vi "PI Measurement Type String Info.vi"(11 "Prompt Measurement Type String":string) -> (0 "Enumerations":string[](array[string]), 1 "Default Value":string, 2 "Is Enum?":bool, 3 "Is Scalar?":bool, 4 "comma list":string, 5 "Units (Scalar)":string)   [LabVIEW 2011]
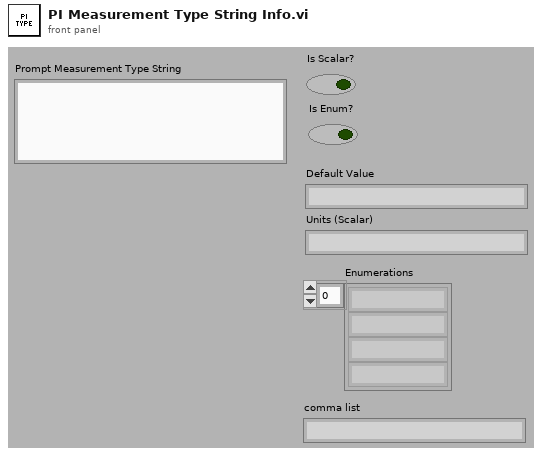
[diagram p1: front panel]
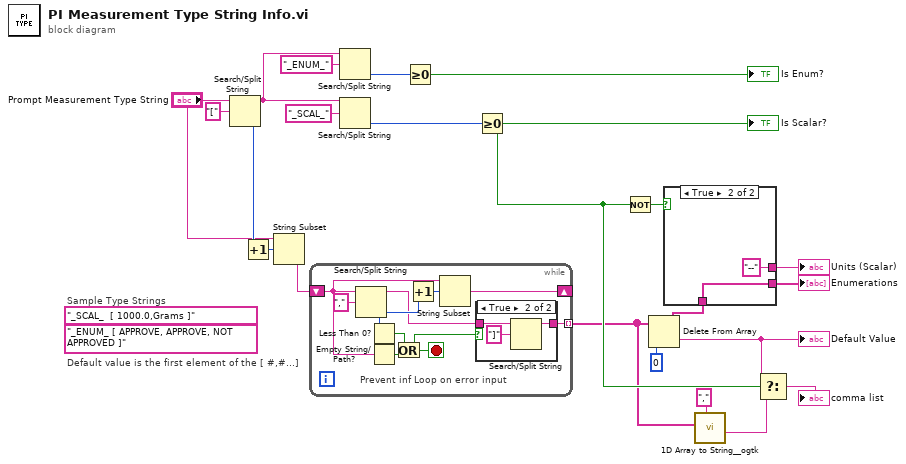
[diagram p0: block diagram]
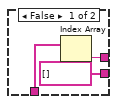
[diagram p2: hidden frame]
diagram:
  (unwired) "_ENUM_ [ APPROVE, APPROVE, NOT APPROVED ]" ("Name")
  (unwired) "_SCAL_  [ 1000.0,Grams ]" ("Name")
  # "Default value is the first element of the [ #,#...]"
  # "Sample Type Strings"
  n1 = Search/Split String(string="Prompt Measurement Type String", search string/char (-)="[") -> (substring before match=w9:string, offset of match=w19:i32)  [unwired: 2 out]
  n2 = Increment(x=w19) -> (x+1=w18:i32)
  n3 = String Subset(string="Prompt Measurement Type String", offset (0)=w18) -> (substring=w17:string)  [unwired: 1 out]
  n4 = while {
    shift-right: [w28] -> _
    shift-left: w17 -> [w26]
    tunnel: [w29] -> w3 mode=indexing
    stop <- w23 stop-if-true
    # "Prevent inf Loop on error input"
    n5 = Search/Split String(string=w26, search string/char (-)=",") -> (substring before match=w27:string, offset of match=w30:i32)  [unwired: 2 out]
    n6 = Less Than 0?(x=w30) -> (x < 0?=w25:bool)
    n7 = Empty String/Path?(string/path=w26) -> (empty?=w24:bool)
    n8 = Or(x=w25, y=w24) -> (x .or. y?=w23:bool)
    n9 = Increment(x=w30) -> (x+1=w31:i32)
    n10 = String Subset(string=w26, offset (0)=w31) -> (substring=w28:string)  [unwired: 1 out]
    n11 = case shown="True" w23 {
      tunnel: w27 -> [w33 w35]
      tunnel: [w33 w34] -> w29
      frame False {
      }
      frame True {
        n12 = Search/Split String(string=w35, search string/char (-)="]") -> (substring before match=w34:string)  [unwired: 3 out]
      }
    }
  }
  n13 = Search/Split String(string=w9, search string/char (-)="_ENUM_") -> (offset of match=w8:i32)  [unwired: 3 out]
  n14 = Search/Split String(string=w9, search string/char (-)="_SCAL_") -> (offset of match=w20:i32)  [unwired: 3 out]
  n15 = Greater Or Equal To 0?(x=w8) -> (x >= 0?=→"Is Enum?":bool)
  n16 = Greater Or Equal To 0?(x=w20) -> (x >= 0?=w6:bool)
  "Is Scalar?" <- w6
  n17 = Not(x=w6) -> (.not. x?=w11:bool)
  n18 = Delete From Array(array=w3, index=0) -> (deleted portion=w5:string, array with subset deleted=w14:string[])  [unwired: 1 in]
  "Default Value" <- w5
  n19 = case shown="True" w11 {
    tunnel: w14 -> [w39 w40]
    tunnel: [w38 "--" ("Prompt Measurement Type String")] -> w13
    tunnel: [string[] [] w40] -> w12
    frame False {
      n20 = Index Array(array=w39) -> (element=w38:string)  [unwired: 1 in]
    }
    frame True {
    }
  }
  "Enumerations" <- w12
  "Units (Scalar)" <- w13
  n21 = call "1D Array to String__ogtk.vi"("delimiter (Tab)"=",", "Array of Strings"=w3) -> ("delimited string"=w2:string)  [unwired: 9 in]
  n22 = Select(t=w5, s=w6, f=w2) -> (s? t:f=→"comma list":string)
